vi "Test Throwing Error.vi"(8 "error in (no error)":errorcluster, 11 "VI Tester Setup Error in":refnum<class "VI Tester Setup Error.lvclass">) -> (0 "error out":errorcluster, 3 "VI Tester Setup Error out":refnum<class "VI Tester Setup Error.lvclass">)   [LabVIEW 2020, in "VI Tester Setup Error.lvclass"]
uses:
  VI Tester Setup Error.lvclass
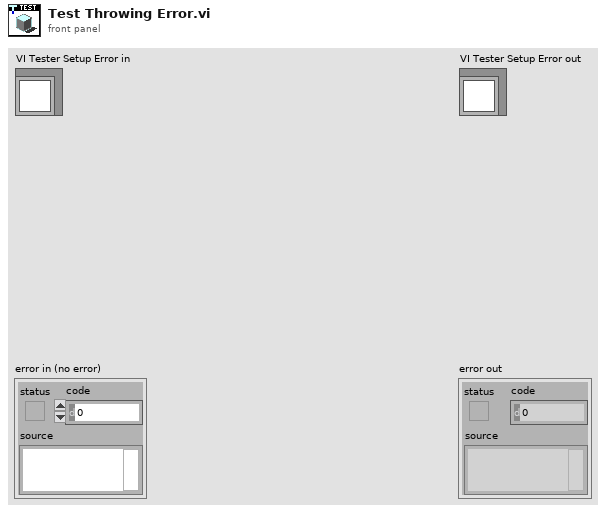
[diagram p1: front panel]
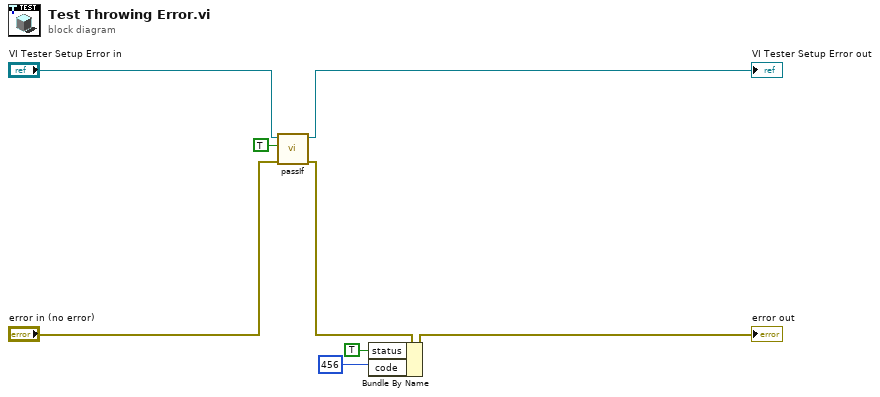
[diagram p0: block diagram]
diagram:
  n1 = call-dynamic "passIf.vi"("error in (no error)"="error in (no error)", "pass"=TRUE, "TestCase in"="VI Tester Setup Error in") -> ("error out"=w2:errorcluster, "TestCase out"=→"VI Tester Setup Error out":refnum<class "VI Tester Setup Error.lvclass">)  [unwired: 7 in]
  n2 = Bundle By Name(cluster=w2, "status"=TRUE, "code"=456) -> (→"error out":errorcluster)
